vi "Read Current Speed.vi"(8 "error in (no error)":errorcluster, 11 "XY Stage Controller in":refnum<class "XY Stage Controller.lvclass">) -> (0 "error out":errorcluster, 1 "Y Current Speed":dbl, 2 "X Current Speed":dbl, 3 "XY Stage Controller out":refnum<class "XY Stage Controller.lvclass">)   [LabVIEW 2022 SP3, in "XY Stage Controller.lvclass"]
uses:
  XY Stage Controller.lvclass
  XY Stage Controller.lvclass/XY Stage Controller.ctl
  XY Stage Data Class/XY Stage Data Class.lvclass/XY Stage Data Class.ctl
  XY Stage Data Class/XY Stage Data Class.lvclass
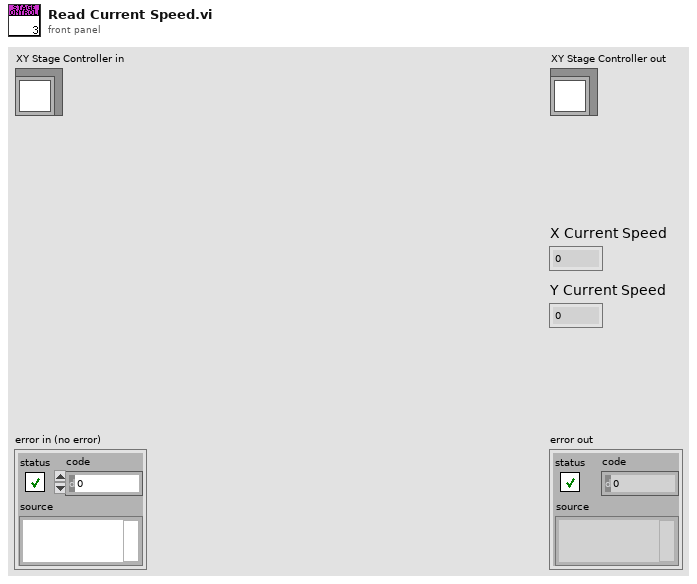
[diagram p1: front panel]
types:
  T1 = typedef "XY Stage Data Class.lvclass/Current Speed.ctl" = cluster{"X Current Speed":dbl, "Y Current Speed":dbl}
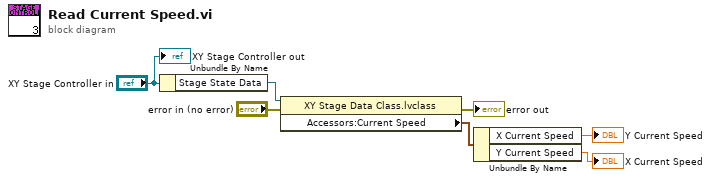
[diagram p0: block diagram]
diagram:
  n1 = Unbundle By Name("XY Stage Controller in") -> ("Stage State Data"=w6:refnum<data-value>)
  n2 = property class="XY Stage Data Class.lvclass"(reference=w6, error in="error in (no error)") -> (error out=→"error out":errorcluster, "Accessors:Current Speed"=w5:T1)  [unwired: 1 out]
  n3 = Unbundle By Name(w5) -> ("X Current Speed"=→"Y Current Speed":dbl, "Y Current Speed"=→"X Current Speed":dbl)
  "XY Stage Controller out" <- "XY Stage Controller in"
